vi "Read Autokey.vi"(8 "error in (no error)":errorcluster, 11 "TypeMap in":refnum<class "TypeMap.lvclass">) -> (0 "error out":errorcluster, 2 "Autokey":string, 3 "TypeMap out":refnum<class "TypeMap.lvclass">)   [LabVIEW 2020, in "ORM.lvlib" / "TypeMap.lvclass"]
uses:
  TypeMap.lvclass
  TypeMap.lvclass/TypeMap.ctl
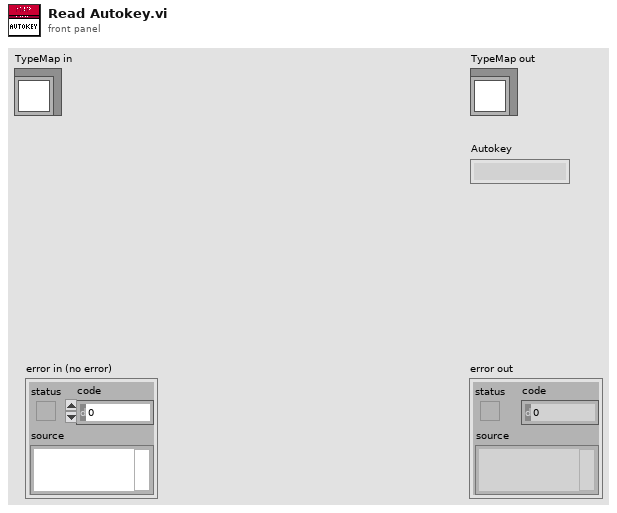
[diagram p1: front panel]
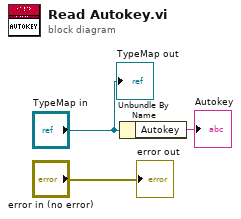
[diagram p0: block diagram]
diagram:
  n1 = Unbundle By Name("TypeMap in") -> ("Autokey"=→"Autokey":string)
  "error out" <- "error in (no error)"
  "TypeMap out" <- "TypeMap in"
